vi "Vicon2JointAngles.vi"(6 "Operation(GetData)":T1, 7 "JointAngleDir([-1,1,1,-1])":dbl[](array[numeric])=[-1.0, 1.0, 1.0, -1.0], 8 "error in (no error)":errorcluster, 9 "LockHipAbduction(F)":bool, 10 "LockHipRotation(T)":bool=TRUE, 11 "ViconIMU in (rad)":dbl[](array[numeric])) -> (0 "error out":errorcluster, 3 "Joint Angles (rad)":dbl[](array[numeric]) format="%#.4f")   [LabVIEW 2016]
uses:
  <vilib>/Analysis/Matrix/Datatypes/RealMatrix.ctl
  TypeDef/IMU_operation.ctl
  <vilib>/Analysis/coordinate.llb/Euler Rotation Order.ctl
  <vilib>/Analysis/BLAS.llb/LV_Transpose.ctl
  Classes/SerialChain/TypeDef/xyzO.ctl
  <vilib>/Analysis/Matrix/Numeric/Conversions/Array To Matrix - RA2.vi
  <vilib>/Analysis/BLAS.llb/dgemm - General Matrix-Matrix Product (DBL).vi
  <vilib>/Analysis/7linalg.llb/Create Special Real Matrix.vi
  <vilib>/Analysis/NI_AALPro.lvlib
  <vilib>/Analysis/NI_AALBLAS.lvlib
  <vilib>/Analysis/Matrix/NI_Matrix.lvlib
  Classes/SerialChain/SerialChain.lvclass
panel:
  out "R_CtoS_Shank":T2 format="%#.3f"
  out "R_CtoS_Thigh":T2 format="%#.3f"
  out "R_CtoS_Hip":T2 format="%#.3f"
  in  "UseStandPos(T)":bool=TRUE
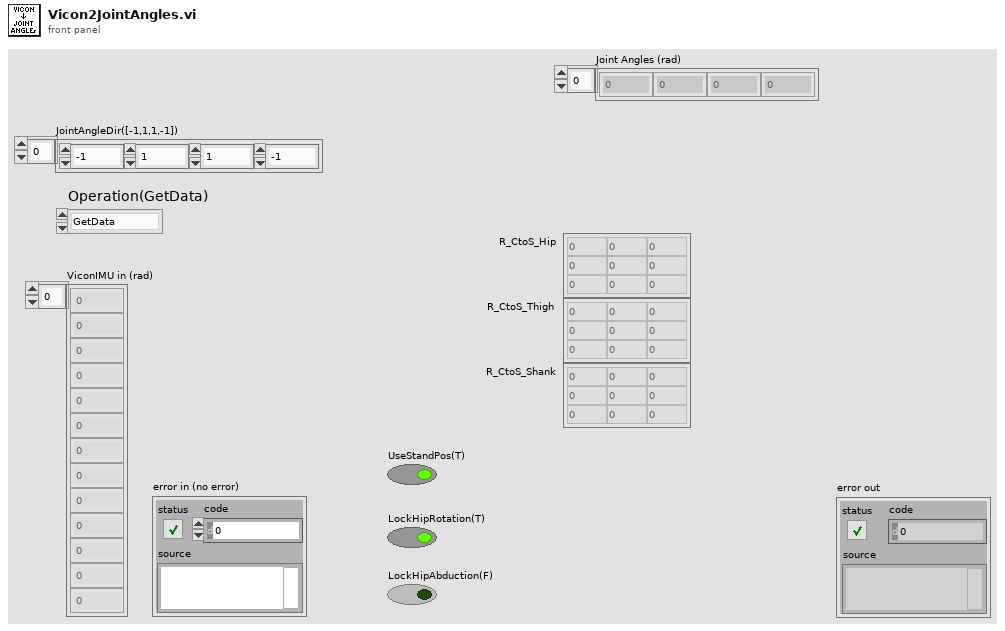
[diagram p1: front panel]
types:
  T1 = typedef "IMU_operation.ctl" = enum16{"GetData", "ClearStandPos", "SetStandPos"}
  T2 = typedef "NI_Matrix.lvlib/RealMatrix.ctl" = dbl[][]
  T3 = typedef "SerialChain.lvclass/xyzO.ctl" = enum16{"X", "Y", "Z", "O"}
  T4 = typedef "NI_AALPro.lvlib/Euler Rotation Order.ctl" = u16
  T5 = typedef "NI_AALBLAS.lvlib/LV_Transpose.ctl" = i32
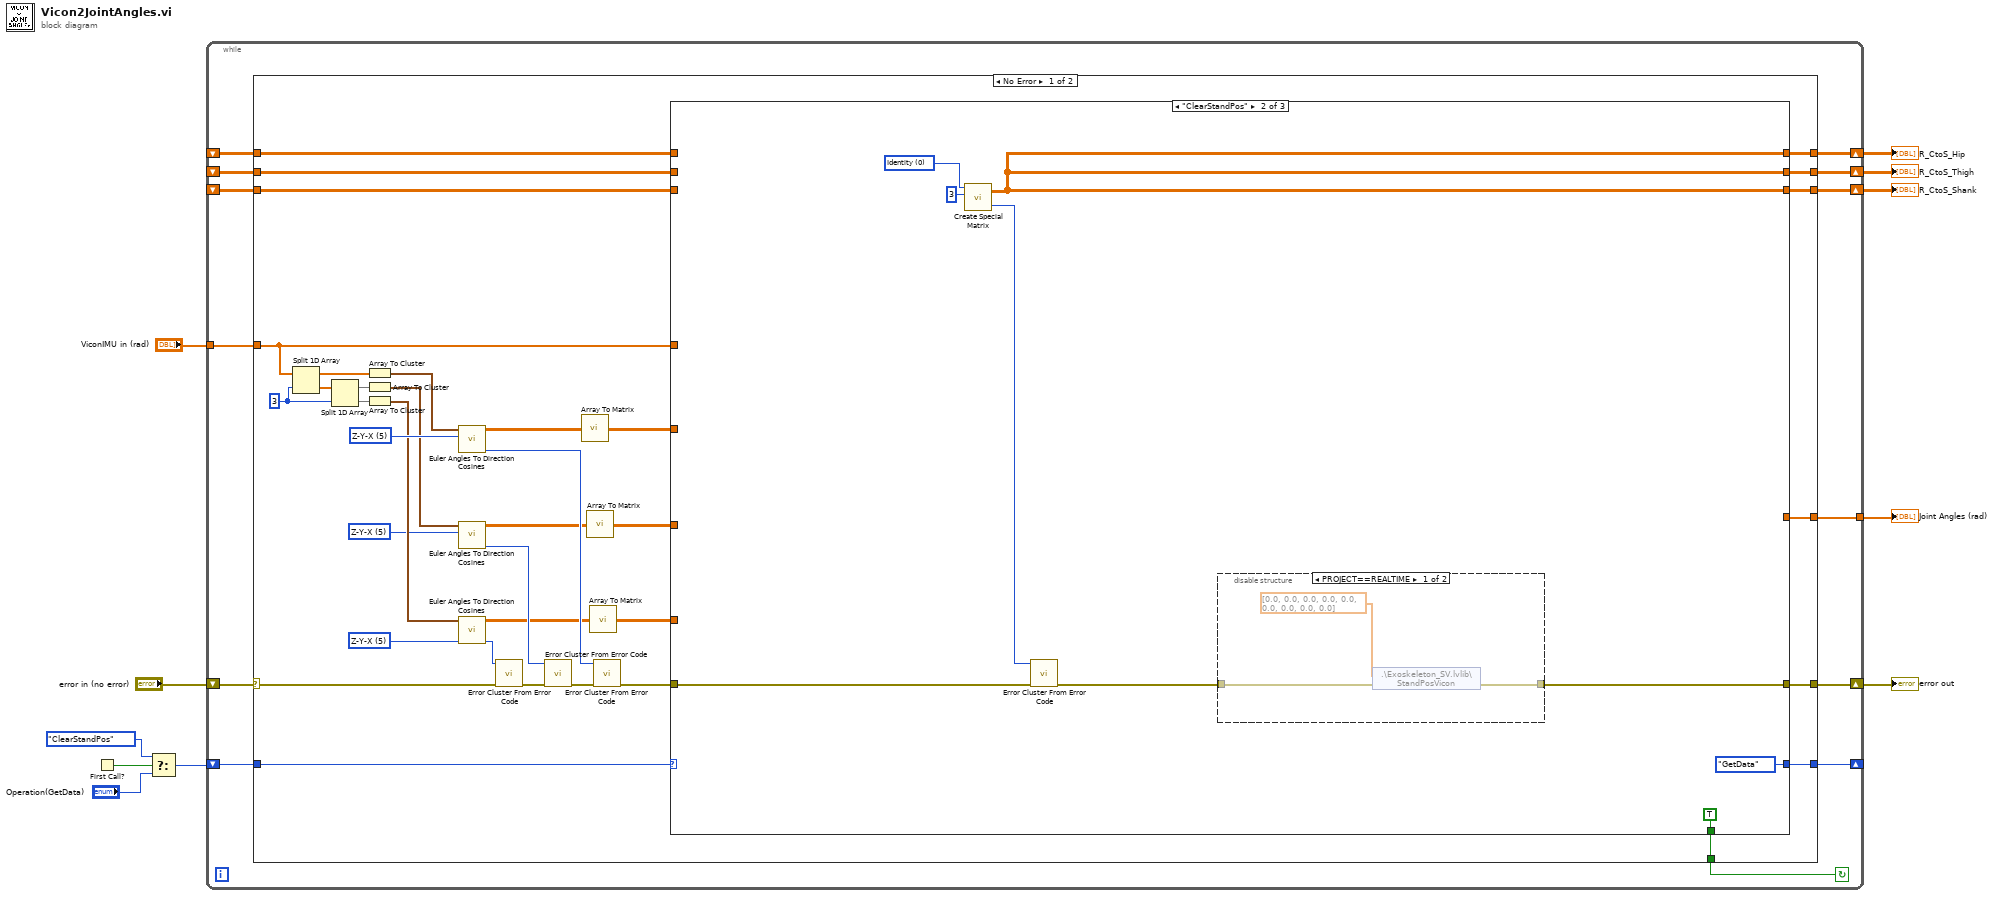
[diagram p0: block diagram]
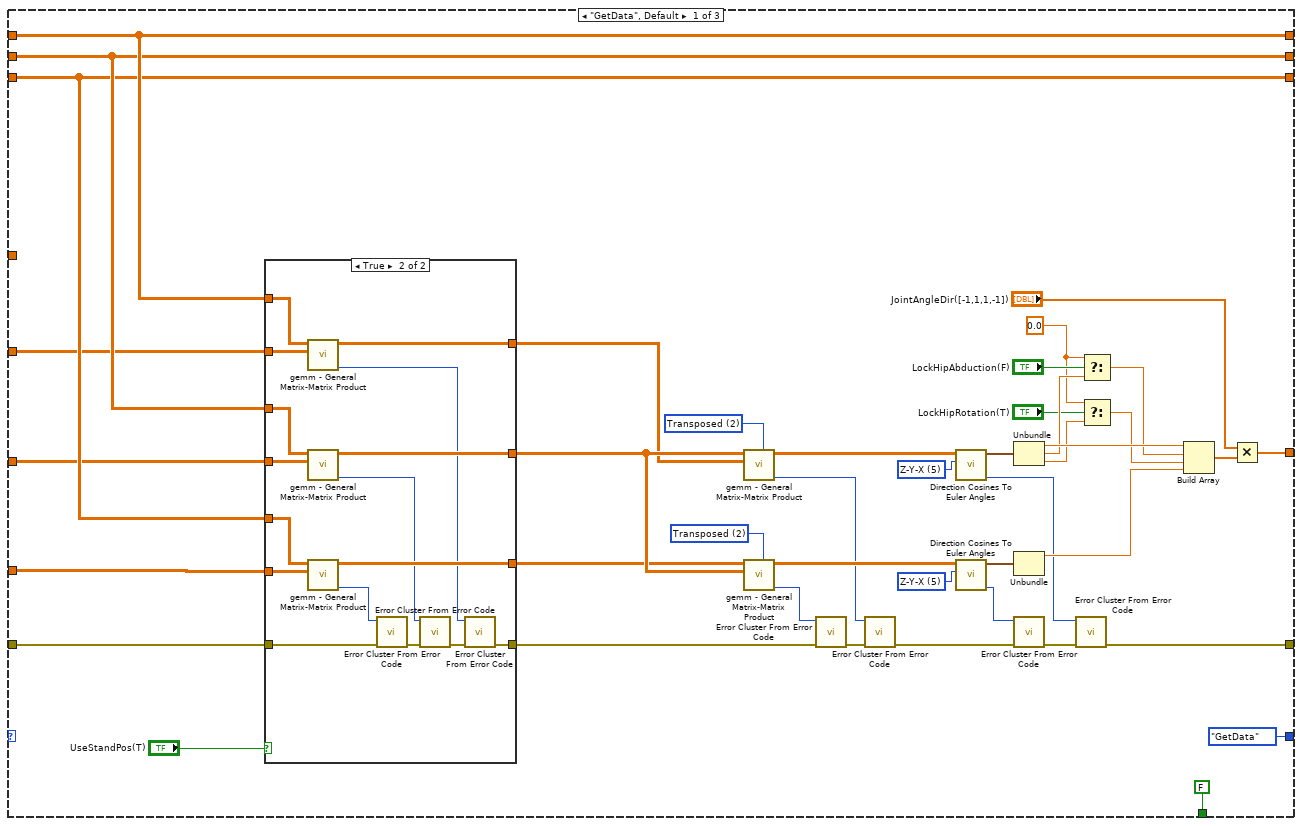
[diagram p2: hidden frame]
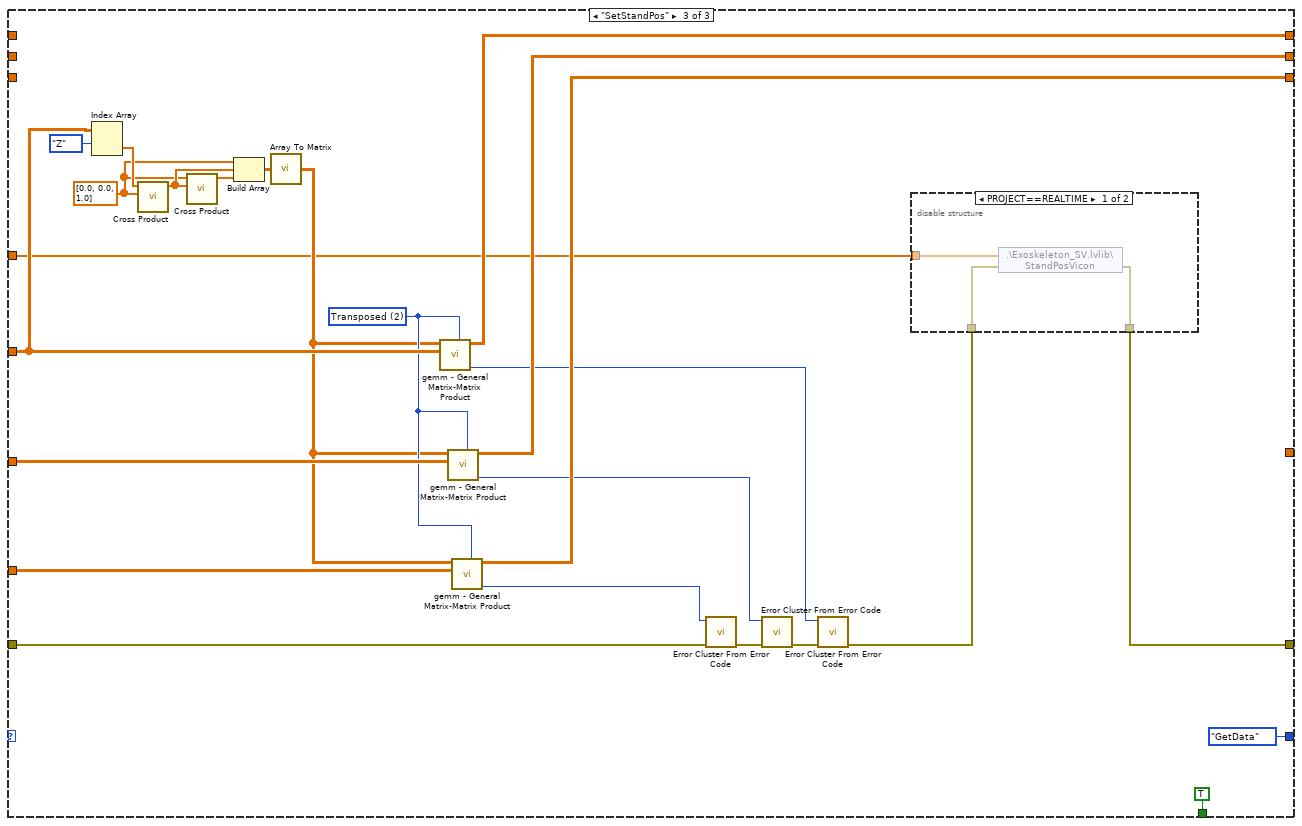
[diagram p5: hidden frame]
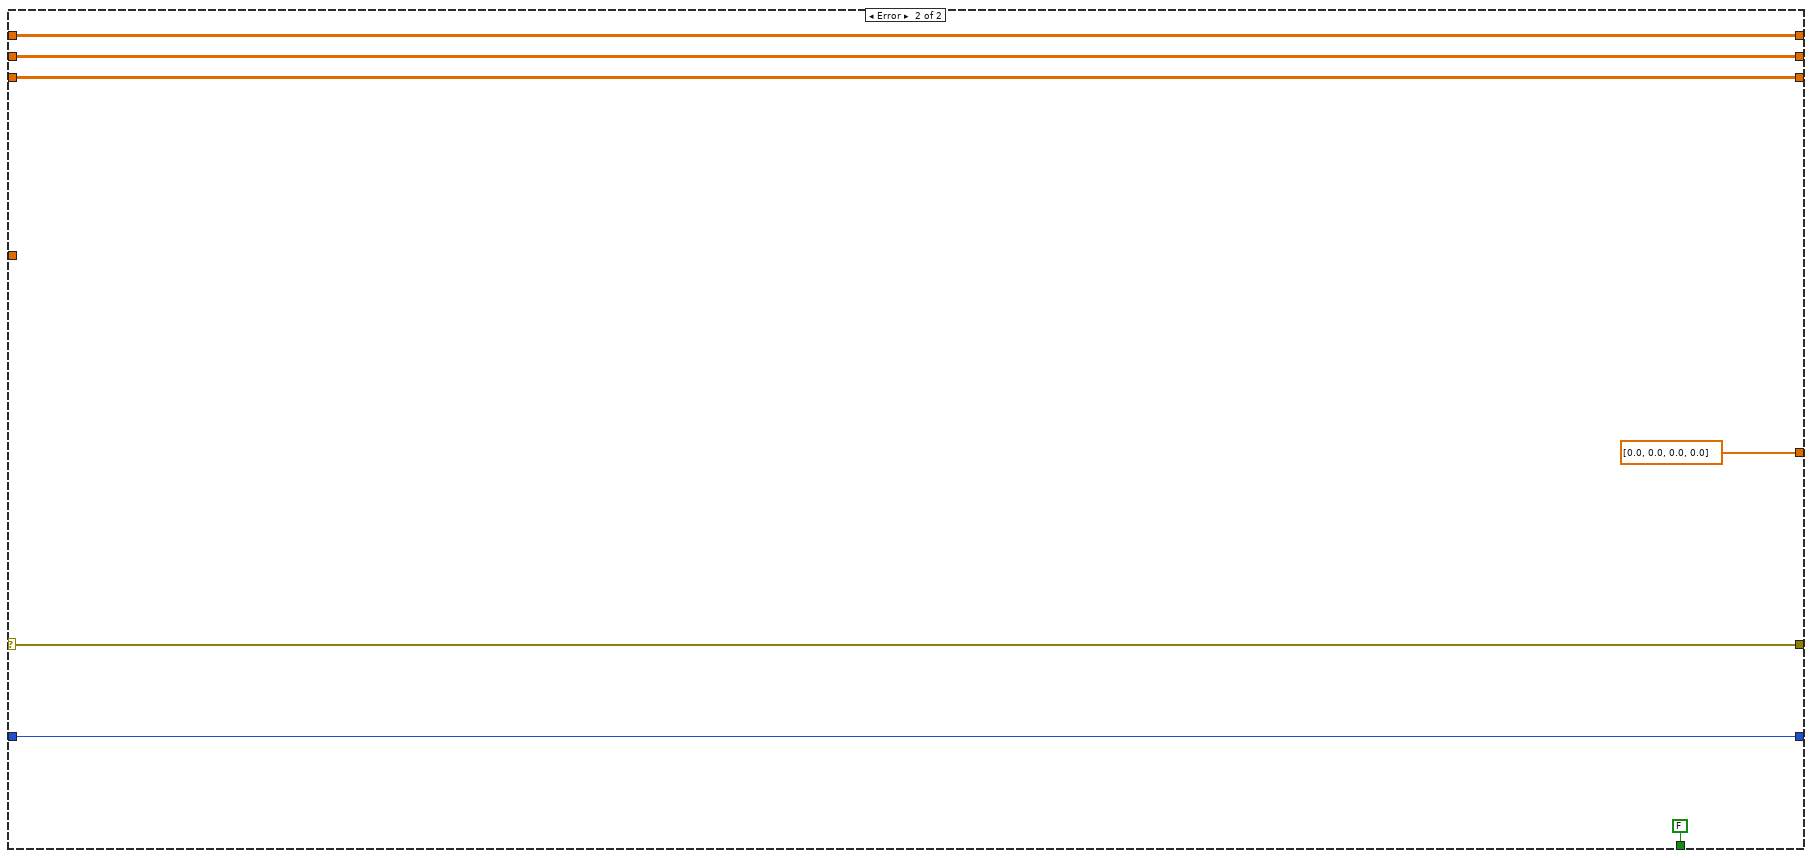
[diagram p7: hidden frame]
diagram:
  n1 = First Call?() -> (First Call?: T/F=w2:bool)
  n2 = Select(t=IMU_operation."ClearStandPos", s=w2, f="Operation(GetData)") -> (s? t:f=w4:T1)
  n3 = while {
    tunnel: [w23] -> w9
    shift-right: [w24] -> w10
    shift-left: "error in (no error)" -> [w22]
    tunnel: "ViconIMU in (rad)" -> [w21]
    shift-right: [w20] -> w7
    shift-left: _ -> [w17]
    shift-right: [w19] -> w6
    shift-left: _ -> [w16]
    shift-right: [w18] -> w5
    shift-left: _ -> [w15]
    shift-right: [w13] -> _
    shift-left: w4 -> [w14]
    stop <- w12 continue-if-true
    n4 = case shown="No Error" w22 {
      selector: w22 -> [w28 w171]
      tunnel: [w60 w171] -> w24
      tunnel: [w59 dbl[] [0.0, 0.0, 0.0, 0.0]] -> w23
      tunnel: w21 -> [w27 _]
      tunnel: [w58 w167] -> w20
      tunnel: [w57 w166] -> w19
      tunnel: [w56 w165] -> w18
      tunnel: w17 -> [w55 w167]
      tunnel: w16 -> [w54 w166]
      tunnel: w15 -> [w53 w165]
      tunnel: w14 -> [w29 w170]
      tunnel: [w26 w170] -> w13
      tunnel: [w25 FALSE] -> w12
      frame No Error {
        w48 = 3 ("index")
        w39 = T4 5 items=["X-Y-Z", "X-Z-Y", "Y-X-Z", "Y-Z-X", "Z-X-Y", "Z-Y-X", "X-Y-X", "X-Z-X", "Y-X-Y", "Y-Z-Y", "Z-X-Z", "Z-Y-Z"] ("rotation order")
        w36 = T4 5 items=["X-Y-Z", "X-Z-Y", "Y-X-Z", "Y-Z-X", "Z-X-Y", "Z-Y-X", "X-Y-X", "X-Z-X", "Y-X-Y", "Y-Z-Y", "Z-X-Z", "Z-Y-Z"] ("rotation order")
        w34 = T4 5 items=["X-Y-Z", "X-Z-Y", "Y-X-Z", "Y-Z-X", "Z-X-Y", "Z-Y-X", "X-Y-X", "X-Z-X", "Y-X-Y", "Y-Z-Y", "Z-X-Z", "Z-Y-Z"] ("rotation order")
        n5 = Split 1D Array(array=w27, index=w48) -> (first subarray=w51:dbl[], second subarray=w47:dbl[])
        n6 = Split 1D Array(array=w47, index=w48) -> (first subarray=w50:dbl[], second subarray=w49:dbl[])
        n7 = Array To Cluster(array=w51) -> (cluster=w38:cluster{"[0]":dbl, "[1]":dbl, "[2]":dbl})
        n8 = Array To Cluster(array=w50) -> (cluster=w35:cluster{"[0]":dbl, "[1]":dbl, "[2]":dbl})
        n9 = Array To Cluster(array=w49) -> (cluster=w37:cluster{"[0]":dbl, "[1]":dbl, "[2]":dbl})
        n10 = call <vilib>:"Euler Angles To Direction Cosines.vi"("rotation order"=w39, "Euler Angles"=w38) -> ("error"=w52:i32, "Direction Cosines"=w42:dbl[][])  [unwired: 8 in]
        n11 = call <vilib>:"Euler Angles To Direction Cosines.vi"("rotation order"=w34, "Euler Angles"=w35) -> ("error"=w45:i32, "Direction Cosines"=w41:dbl[][])  [unwired: 8 in]
        n12 = call <vilib>:"Euler Angles To Direction Cosines.vi"("rotation order"=w36, "Euler Angles"=w37) -> ("error"=w46:i32, "Direction Cosines"=w40:dbl[][])  [unwired: 8 in]
        n13 = call <vilib>:"Error Cluster From Error Code.vi"("error in (no error)"=w28, "error code (0)"=w46) -> ("error out"=w43:errorcluster)  [unwired: 7 in]
        n14 = call <vilib>:"Error Cluster From Error Code.vi"("error in (no error)"=w43, "error code (0)"=w45) -> ("error out"=w44:errorcluster)  [unwired: 7 in]
        n15 = call-poly <vilib>:"Array To Matrix.vi"("Real 2D Array"=w42) -> ("Real Matrix"=w30:T2)
        n16 = call-poly <vilib>:"Array To Matrix.vi"("Real 2D Array"=w41) -> ("Real Matrix"=w31:T2)
        n17 = call-poly <vilib>:"Array To Matrix.vi"("Real 2D Array"=w40) -> ("Real Matrix"=w32:T2)
        n18 = call <vilib>:"Error Cluster From Error Code.vi"("error in (no error)"=w44, "error code (0)"=w52) -> ("error out"=w33:errorcluster)  [unwired: 7 in]
        n19 = case shown="\"ClearStandPos\"" w29 {
          tunnel: [w88 w126 w138] -> w60
          tunnel: [w87 _ _] -> w59
          tunnel: [w82 w123 w151] -> w58
          tunnel: [w81 w123 w150] -> w57
          tunnel: [w80 w123 w149] -> w56
          tunnel: w55 -> [w82 _ _]
          tunnel: w54 -> [w81 _ _]
          tunnel: w53 -> [w80 _ _]
          tunnel: w33 -> [w79 w128 w142]
          tunnel: w32 -> [w78 _ w153]
          tunnel: w31 -> [w77 _ w154]
          tunnel: w30 -> [w76 _ w152]
          tunnel: w27 -> [_ _ w140]
          tunnel: [IMU_operation."GetData" ("Operation(GetData)") IMU_operation."GetData" ("Operation(GetData)") IMU_operation."GetData" ("Operation(GetData)")] -> w26
          tunnel: [FALSE TRUE TRUE] -> w25
          frame "GetData", Default {
            w63 = 0.0 ("t")
            w73 = T4 5 items=["X-Y-Z", "X-Z-Y", "Y-X-Z", "Y-Z-X", "Z-X-Y", "Z-Y-X", "X-Y-X", "X-Z-X", "Y-X-Y", "Y-Z-Y", "Z-X-Z", "Z-Y-Z"] ("rotation order")
            w75 = T4 5 items=["X-Y-Z", "X-Z-Y", "Y-X-Z", "Y-Z-X", "Z-X-Y", "Z-Y-X", "X-Y-X", "X-Z-X", "Y-X-Y", "Y-Z-Y", "Z-X-Z", "Z-Y-Z"] ("rotation order")
            w96 = T5 2 items=["Direct", "Conjugated & Transposed", "Transposed"] ("operation B")
            w95 = T5 2 items=["Direct", "Conjugated & Transposed", "Transposed"] ("operation B")
            n20 = case shown="True" "UseStandPos(T)" {
              tunnel: w76 -> [w106 w107]
              tunnel: [w106 w122] -> w83
              tunnel: [w105 w121] -> w94
              tunnel: w77 -> [w105 w118]
              tunnel: w78 -> [w104 w120]
              tunnel: [w104 w119] -> w93
              tunnel: w82 -> [_ w114]
              tunnel: w81 -> [_ w113]
              tunnel: w80 -> [_ w112]
              tunnel: w79 -> [w103 w111]
              tunnel: [w103 w108] -> w91
              frame False {
              }
              frame True {
                n21 = call-poly <vilib>:"gemm - General Matrix-Matrix Product.vi"("B"=w107, "A"=w114) -> ("error"=w117:i32, "dgemm"=w122:T2)  [unwired: 8 in]
                n22 = call-poly <vilib>:"gemm - General Matrix-Matrix Product.vi"("B"=w118, "A"=w113) -> ("error"=w116:i32, "dgemm"=w121:T2)  [unwired: 8 in]
                n23 = call-poly <vilib>:"gemm - General Matrix-Matrix Product.vi"("B"=w120, "A"=w112) -> ("error"=w115:i32, "dgemm"=w119:T2)  [unwired: 8 in]
                n24 = call <vilib>:"Error Cluster From Error Code.vi"("error in (no error)"=w111, "error code (0)"=w115) -> ("error out"=w110:errorcluster)  [unwired: 7 in]
                n25 = call <vilib>:"Error Cluster From Error Code.vi"("error in (no error)"=w110, "error code (0)"=w116) -> ("error out"=w109:errorcluster)  [unwired: 7 in]
                n26 = call <vilib>:"Error Cluster From Error Code.vi"("error in (no error)"=w109, "error code (0)"=w117) -> ("error out"=w108:errorcluster)  [unwired: 7 in]
              }
            }
            n27 = call-poly <vilib>:"gemm - General Matrix-Matrix Product.vi"("operation B"=w96, "B"=w83, "A"=w94) -> ("error"=w90:i32, "dgemm"=w97:T2)  [unwired: 7 in]
            n28 = call-poly <vilib>:"gemm - General Matrix-Matrix Product.vi"("operation B"=w95, "B"=w94, "A"=w93) -> ("error"=w89:i32, "dgemm"=w100:T2)  [unwired: 7 in]
            n29 = call <vilib>:"Error Cluster From Error Code.vi"("error in (no error)"=w91, "error code (0)"=w89) -> ("error out"=w86:errorcluster)  [unwired: 7 in]
            n30 = call <vilib>:"Error Cluster From Error Code.vi"("error in (no error)"=w86, "error code (0)"=w90) -> ("error out"=w85:errorcluster)  [unwired: 7 in]
            n31 = call <vilib>:"Direction Cosines To Euler Angles.vi"("rotation order"=w73, "Direction Cosines"=w97) -> ("error"=w71:i32, "Euler Angles"=w72:cluster{"phi":dbl, "theta":dbl, "psi":dbl})  [unwired: 8 in]
            n32 = call <vilib>:"Direction Cosines To Euler Angles.vi"("rotation order"=w75, "Direction Cosines"=w100) -> ("error"=w70:i32, "Euler Angles"=w74:cluster{"phi":dbl, "theta":dbl, "psi":dbl})  [unwired: 8 in]
            n33 = Unbundle(w72) -> ("phi"=w99:dbl, "theta"=w67:dbl, "psi"=w64:dbl)
            n34 = Unbundle(w74) -> ("phi"=w98:dbl)  [unwired: 2 out]
            n35 = call <vilib>:"Error Cluster From Error Code.vi"("error in (no error)"=w85, "error code (0)"=w70) -> ("error out"=w69:errorcluster)  [unwired: 7 in]
            n36 = call <vilib>:"Error Cluster From Error Code.vi"("error in (no error)"=w69, "error code (0)"=w71) -> ("error out"=w88:errorcluster)  [unwired: 7 in]
            n37 = Select(t=w63, s="LockHipAbduction(F)", f=w67) -> (s? t:f=w84:dbl)
            n38 = Select(t=w63, s="LockHipRotation(T)", f=w64) -> (s? t:f=w65:dbl)
            n39 = Build Array(w99, w84, w65, w98) -> (w102:dbl[])
            n40 = Multiply(x="JointAngleDir([-1,1,1,-1])", y=w102) -> (x*y=w87:dbl[])
          }
          frame "ClearStandPos" {
            w130 = 0 items=["Identity", "Diagonal", "Toeplitz", "Vandermonde", "Companion", "Hankel", "Hadamard", "Wilkinson", "Hilbert", "Inverse Hilbert", "Rosser", "Pascal"] ("matrix type")
            n41 = call-poly <vilib>:"Create Special Matrix.vi"("matrix type"=w130, "matrix size"=3) -> ("Special Matrix"=w123:T2, "error"=w129:i32)  [unwired: 3 in]
            n42 = call <vilib>:"Error Cluster From Error Code.vi"("error in (no error)"=w128, "error code (0)"=w129) -> ("error out"=w127:errorcluster)  [unwired: 7 in]
            n43 = disable-structure shown="PROJECT==REALTIME" {
              disable-tunnel: w127 -> [w133 w135]
              disable-tunnel: [w132 w135] -> w126
              frame condition #0 {
                n44 = shared-variable ".\\Exoskeleton_SV.lvlib\\StandPosVicon"(dbl[] [0.0, 0.0, 0.0, 0.0, 0.0, 0.0, 0.0, 0.0, 0.0] ("ZeroOrient 2"), error in=w133) -> (error out=w132:errorcluster)
              }
              frame condition #1 (active) {
              }
            }
          }
          frame "SetStandPos" {
            w148 = T5 2 items=["Direct", "Conjugated & Transposed", "Transposed"] ("operation B")
            w155 = dbl[] [0.0, 0.0, 1.0]
            n45 = Index Array(array=w152, index (row)=xyzO."Z" ("XYZ")) -> (element=w158:dbl[])  [unwired: 1 in]
            n46 = call <vilib>:"Cross Product.vi"("B Vector"=w155, "A Vector"=w158) -> ("Cross Product"=w157:dbl[])  [unwired: 8 in, 1 out]
            n47 = call <vilib>:"Cross Product.vi"("B Vector"=w157, "A Vector"=w155) -> ("Cross Product"=w156:dbl[])  [unwired: 8 in, 1 out]
            n48 = Build Array(w155, w157, w156) -> (w160:dbl[][])
            n49 = call-poly <vilib>:"Array To Matrix.vi"("Real 2D Array"=w160) -> ("Real Matrix"=w141:T2)
            n50 = call-poly <vilib>:"gemm - General Matrix-Matrix Product.vi"("operation B"=w148, "B"=w152, "A"=w141) -> ("error"=w143:i32, "dgemm"=w151:T2)  [unwired: 7 in]
            n51 = call-poly <vilib>:"gemm - General Matrix-Matrix Product.vi"("operation B"=w148, "B"=w154, "A"=w141) -> ("error"=w144:i32, "dgemm"=w150:T2)  [unwired: 7 in]
            n52 = call-poly <vilib>:"gemm - General Matrix-Matrix Product.vi"("operation B"=w148, "B"=w153, "A"=w141) -> ("error"=w145:i32, "dgemm"=w149:T2)  [unwired: 7 in]
            n53 = call <vilib>:"Error Cluster From Error Code.vi"("error in (no error)"=w142, "error code (0)"=w145) -> ("error out"=w147:errorcluster)  [unwired: 7 in]
            n54 = call <vilib>:"Error Cluster From Error Code.vi"("error in (no error)"=w147, "error code (0)"=w144) -> ("error out"=w146:errorcluster)  [unwired: 7 in]
            n55 = call <vilib>:"Error Cluster From Error Code.vi"("error in (no error)"=w146, "error code (0)"=w143) -> ("error out"=w139:errorcluster)  [unwired: 7 in]
            n56 = disable-structure shown="PROJECT==REALTIME" {
              disable-tunnel: w140 -> [w163 _]
              disable-tunnel: w139 -> [w162 w164]
              disable-tunnel: [w161 w164] -> w138
              frame condition #0 {
                n57 = shared-variable ".\\Exoskeleton_SV.lvlib\\StandPosVicon"(w163, error in=w162) -> (error out=w161:errorcluster)
              }
              frame condition #1 (active) {
              }
            }
          }
        }
      }
      frame Error {
      }
    }
  }
  "Joint Angles (rad)" <- w9
  "error out" <- w10
  "R_CtoS_Shank" <- w5
  "R_CtoS_Hip" <- w7
  "R_CtoS_Thigh" <- w6
